vi "GaussianKernel5x5.vi"() -> ()   [LabVIEW 2022 SP3]
panel:
  out "appended array":dbl[][](array[numeric])
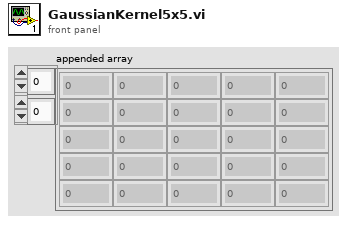
[diagram p1: front panel]
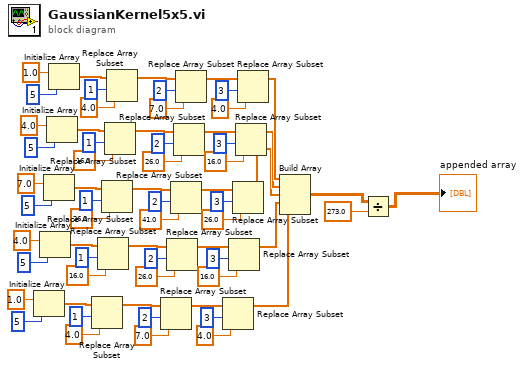
[diagram p0: block diagram]
diagram:
  n1 = Initialize Array(1.0 ("element"), 5 ("dimension size")) -> (w15:dbl[])
  n2 = Initialize Array(4.0 ("element"), 5 ("dimension size")) -> (w26:dbl[])
  n3 = Initialize Array(7.0 ("element"), 5 ("dimension size")) -> (w37:dbl[])
  n4 = Initialize Array(4.0 ("element"), 5 ("dimension size")) -> (w48:dbl[])
  n5 = Initialize Array(1.0 ("element"), 5 ("dimension size")) -> (w59:dbl[])
  n6 = Replace Array Subset(array=w15, new element=4.0 ("new element/subarray"), index=1) -> (w14:dbl[])
  n7 = Replace Array Subset(array=w26, new element=16.0 ("new element/subarray"), index=1) -> (w25:dbl[])
  n8 = Replace Array Subset(array=w37, new element=26.0 ("new element/subarray"), index=1) -> (w36:dbl[])
  n9 = Replace Array Subset(array=w48, new element=16.0 ("new element/subarray"), index=1) -> (w47:dbl[])
  n10 = Replace Array Subset(array=w59, new element=4.0 ("new element/subarray"), index=1) -> (w58:dbl[])
  n11 = Replace Array Subset(array=w14, new element=7.0 ("new element/subarray"), index=2) -> (w11:dbl[])
  n12 = Replace Array Subset(array=w25, new element=26.0 ("new element/subarray"), index=2) -> (w22:dbl[])
  n13 = Replace Array Subset(array=w36, new element=41.0 ("new element/subarray"), index=2) -> (w33:dbl[])
  n14 = Replace Array Subset(array=w47, new element=26.0 ("new element/subarray"), index=2) -> (w44:dbl[])
  n15 = Replace Array Subset(array=w58, new element=7.0 ("new element/subarray"), index=2) -> (w55:dbl[])
  n16 = Replace Array Subset(array=w11, new element=4.0 ("new element/subarray"), index=3) -> (w4:dbl[])
  n17 = Replace Array Subset(array=w22, new element=16.0 ("new element/subarray"), index=3) -> (w5:dbl[])
  n18 = Replace Array Subset(array=w33, new element=26.0 ("new element/subarray"), index=3) -> (w6:dbl[])
  n19 = Replace Array Subset(array=w44, new element=16.0 ("new element/subarray"), index=3) -> (w7:dbl[])
  n20 = Replace Array Subset(array=w55, new element=4.0 ("new element/subarray"), index=3) -> (w8:dbl[])
  n21 = Build Array(w8, w7, w6, w5, w4) -> (w2:dbl[][])
  n22 = Divide(x=w2, y=273.0) -> (x/y=→"appended array":dbl[][])
